vi "远程中止VI.vi"() -> ()   [LabVIEW 2013]
panel:
  out "错误输出":errorcluster
  out "VI引用":refnum<vi>
  in  "停止按钮":bool
  in  "VI路径":path
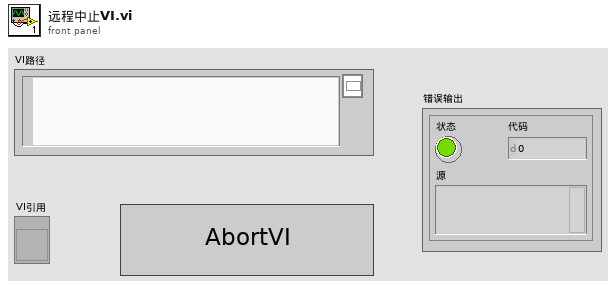
[diagram p1: front panel]
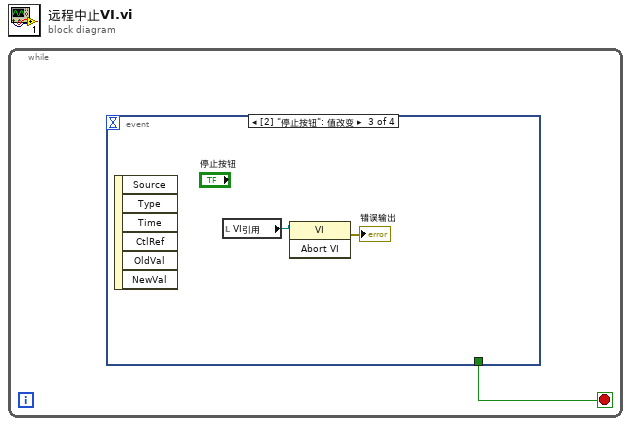
[diagram p0: block diagram]
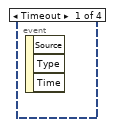
[diagram p2: hidden frame]
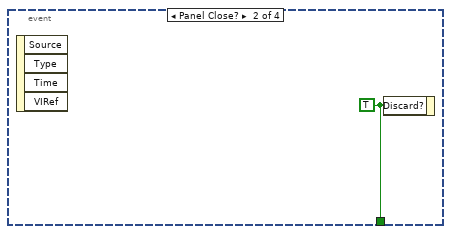
[diagram p3: hidden frame]
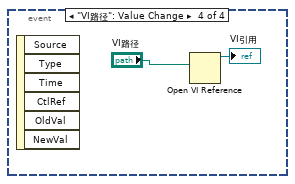
[diagram p4: hidden frame]
diagram:
  n1 = while {
    stop <- w1 stop-if-true
    n2 = event shown="[2] \"停止按钮\": 值改变" {
      selector: _ -> [_ _ _ _]
      dyn-events: _ -> [_ _ _ _]
      timeout: _ -> [_ _ _ _]
      tunnel: [_ w2 _ _] -> w1
      event Timeout {
        n3 = event-data() -> ()  [unwired: 1 in, 3 out]
      }
      event Panel Close? {
        w2 = TRUE ("放弃？")
        n4 = event-data() -> ()  [unwired: 1 in, 4 out]
        n5 = event-data("Discard?"=w2) -> ()  [unwired: 1 in, 1 out]
      }
      event "停止按钮": Value Change {
        n6 = event-data() -> ()  [unwired: 1 in, 6 out]
        n7 = local read "VI引用"() -> (w4:refnum<vi>)
        n8 = invoke class="VI" method="Abort VI"(reference=w4) -> (error out=→"错误输出":errorcluster)  [unwired: 2 in, 2 out]
      }
      event "VI路径": Value Change {
        n9 = event-data() -> ()  [unwired: 1 in, 6 out]
        n10 = Open VI Reference(vi path="VI路径") -> (vi reference=→"VI引用":refnum<vi>)  [unwired: 5 in, 1 out]
      }
    }
  }
